vi "Read value.vi"(8 "error in (no error)":errorcluster, 11 "ServoDatatype in":refnum<class "ServoDatatype.lvclass">) -> (0 "error out":errorcluster, 2 "value":string, 3 "ServoDatatype out":refnum<class "ServoDatatype.lvclass">)   [LabVIEW 2014, in "LabVIEW Universal Trasncriptor Servo.lvlib" / "ServoDatatype.lvclass"]
uses:
  ServoDatatype.lvclass
  ServoDatatype.lvclass/ServoDatatype.ctl
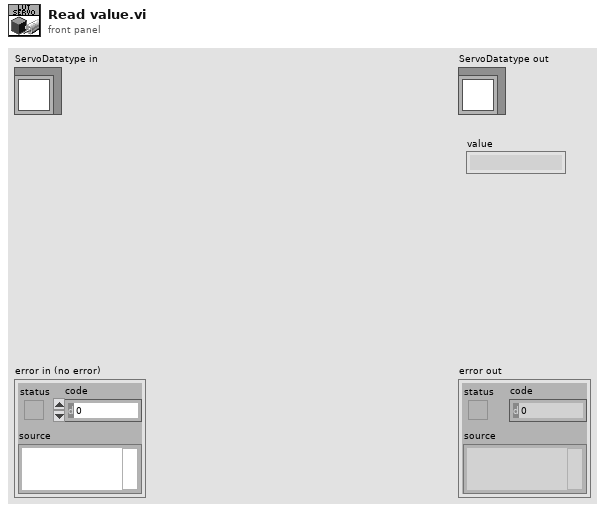
[diagram p1: front panel]
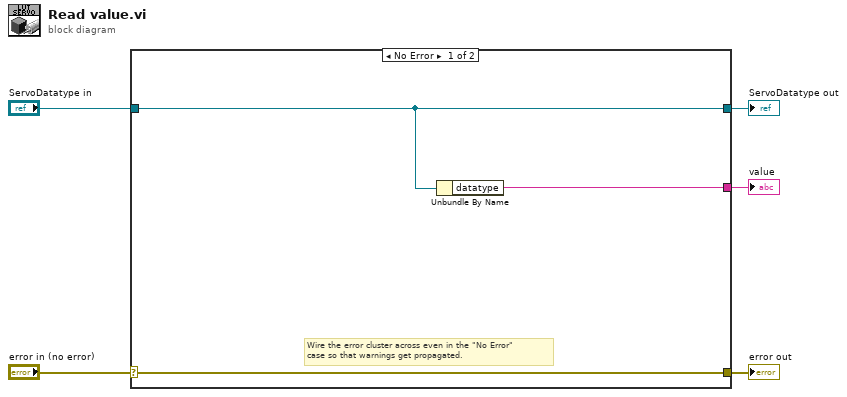
[diagram p0: block diagram]
diagram:
  n1 = case shown="No Error" "error in (no error)" {
    selector: "error in (no error)" -> [w8 w10]
    tunnel: [w8 w10] -> w4
    tunnel: [w7 w9] -> w2
    tunnel: "ServoDatatype in" -> [w7 w9]
    tunnel: [w6 _] -> w1
    frame No Error {
      # "Wire the error cluster across even in the \"No Error\"\ncase so that warnings get propagated."
      n2 = Unbundle By Name(w7) -> ("datatype"=w6:string)
    }
    frame Error {
    }
  }
  "error out" <- w4
  "ServoDatatype out" <- w2
  "value" <- w1
